vi "Run.vi"(8 "error in (no error)":errorcluster, 11 "TCS in":refnum<class "TCS.lvclass">) -> (0 "error out":errorcluster, 3 "TCS out":refnum<class "TCS.lvclass">)   [LabVIEW 2018, in "TCS.lvclass"]
uses:
  TCS.lvclass
  TCS.lvclass/TCS.ctl
  State Machine/State Machine.lvclass
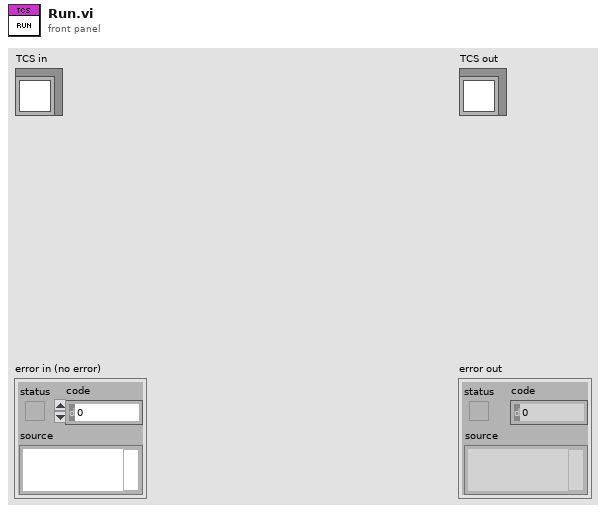
[diagram p1: front panel]
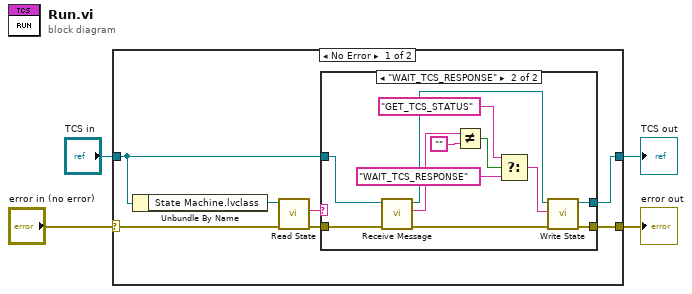
[diagram p0: block diagram]
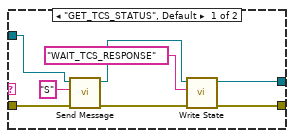
[diagram p2: hidden frame]
diagram:
  n1 = case shown="No Error" "error in (no error)" {
    selector: "error in (no error)" -> [w8 w33]
    tunnel: [w6 w33] -> w2
    tunnel: [w7 w32] -> w1
    tunnel: "TCS in" -> [w5 w32]
    frame No Error {
      n2 = Unbundle By Name(w5) -> ("State Machine.lvclass"=w11:refnum<class "State Machine.lvclass">)
      n3 = call-dynamic "Read State.vi"("error in (no error)"=w8, "State Machine in"=w11) -> ("error out"=w9:errorcluster, "State"=w10:string)  [unwired: 7 in, 1 out]
      n4 = case shown="\"WAIT_TCS_RESPONSE\"" w10 {
        tunnel: w9 -> [w16 w27]
        tunnel: [w19 w24] -> w7
        tunnel: [w18 w22] -> w6
        tunnel: w5 -> [w12 w20]
        frame "GET_TCS_STATUS", Default {
          n5 = call "Send Message.vi"("error in (no error)"=w16, "message"="S", "TCS in"=w12) -> ("error out"=w17:errorcluster, "TCS out"=w13:refnum<class "TCS.lvclass">)  [unwired: 7 in]
          n6 = call "Write State.vi"("error in (no error)"=w17, "State"="WAIT_TCS_RESPONSE" ("message"), "TCS in"=w13) -> ("error out"=w18:errorcluster, "TCS out"=w19:refnum<class "TCS.lvclass">)  [unwired: 7 in]
        }
        frame "WAIT_TCS_RESPONSE" {
          n7 = call "Receive Message.vi"("error in (no error)"=w27, "TCS in"=w20) -> ("error out"=w21:errorcluster, "Rx message"=w26:string, "TCS out"=w25:refnum<class "TCS.lvclass">)  [unwired: 7 in]
          n8 = Not Equal?(x=w26, y="") -> (x != y?=w30:bool)
          n9 = Select(t="GET_TCS_STATUS", s=w30, f="WAIT_TCS_RESPONSE") -> (s? t:f=w23:string)
          n10 = call "Write State.vi"("error in (no error)"=w21, "State"=w23, "TCS in"=w25) -> ("error out"=w22:errorcluster, "TCS out"=w24:refnum<class "TCS.lvclass">)  [unwired: 7 in]
        }
      }
    }
    frame Error {
    }
  }
  "error out" <- w2
  "TCS out" <- w1
